vi "decimate_waveforms.vi"(6 "decimating factor":i32=1, 7 "averaging":bool, 8 "error in (no error)":errorcluster, 11 "Input Signal":waveform(dbl)[](array[waveform])) -> (0 "error out":errorcluster, 3 "Decimated Waveforms":waveform(dbl)[](array[waveform]))   [LabVIEW 2016]
doc: "Decimates the input sequence X by the decimating factor and the averaging Boolean control."
uses:
  <vilib>/Analysis/2dsp.llb/Decimate (single shot, DBL).vi
  <vilib>/Analysis/NI_AALPro.lvlib
panel:
  # "by Marco Tedaldi, Brain Research Institute, University of Zurich, 2013"
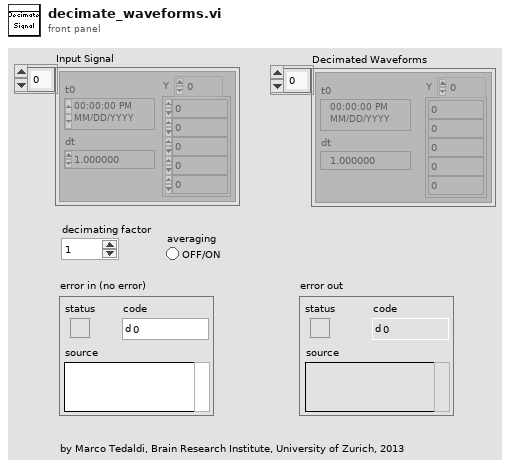
[diagram p1: front panel]
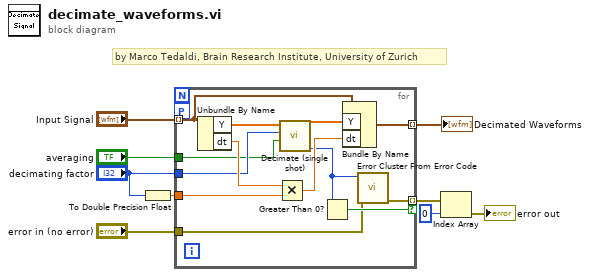
[diagram p0: block diagram]
diagram:
  # "by Marco Tedaldi, Brain Research Institute, University of Zurich"
  n1 = To Double Precision Float(number="decimating factor") -> (double precision float=w7:dbl)
  n2 = for {
    tunnel: "Input Signal" -> [w21] mode=indexing
    tunnel: [w19] -> w6 mode=indexing
    tunnel: w7 -> [w17]
    tunnel: "decimating factor" -> [w16]
    tunnel: "averaging" -> [w14]
    workers-P: _ -> [_]
    tunnel: "error in (no error)" -> [w12]
    tunnel: [w11] -> w3 mode=indexing if=w13
    n3 = Unbundle By Name(w21) -> ("Y"=w22:dbl[], "dt"=w18:dbl)
    n4 = Multiply(x=w18, y=w17) -> (x*y=w15:dbl)
    n5 = call-poly <vilib>:"Decimate (single shot).vi"("averaging"=w14, "decimating factor"=w16, "X"=w22) -> ("error"=w10:i32, "Decimated Array"=w20:dbl[])  [unwired: 7 in]
    n6 = Greater Than 0?(x=w10) -> (x > 0?=w13:bool)
    n7 = Bundle By Name(cluster=w21, "Y"=w20, "dt"=w15) -> (w19:waveform(dbl))
    n8 = call <vilib>:"Error Cluster From Error Code.vi"("error in (no error)"=w12, "error code (0)"=w10) -> ("error out"=w11:errorcluster)  [unwired: 7 in]
  }
  "Decimated Waveforms" <- w6
  n9 = Index Array(array=w3, index=0) -> (element=→"error out":errorcluster)
